vi "Replace with Caller if Empty.vi"(10 "Test VI (caller) in":string) -> (2 "Test VI (caller) out":string)   [LabVIEW 2020, in "Approval Tests.lvlib"]
uses:
  Approval Tests.lvlib
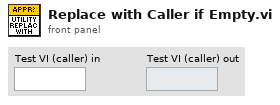
[diagram p1: front panel]
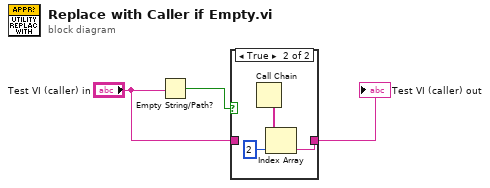
[diagram p0: block diagram]
diagram:
  n1 = Empty String/Path?(string/path="Test VI (caller) in") -> (empty?=w1:bool)
  n2 = case shown="True" w1 {
    tunnel: "Test VI (caller) in" -> [w4 _]
    tunnel: [w4 w7] -> w3
    frame False {
    }
    frame True {
      n3 = Call Chain() -> (call chain=w5:string[])
      n4 = Index Array(array=w5, index=2) -> (element=w7:string)
    }
  }
  "Test VI (caller) out" <- w3
